vi "DO Close.vi"(8 "error in (no error)":errorcluster, 11 "Mech Pump in":refnum<class "Mech Pump.lvclass">) -> (0 "error out":errorcluster)   [LabVIEW 2021, in "Mech Pump.lvlib" / "Mech Pump.lvclass"]
uses:
  Mech Pump.lvclass
  Mech Pump.lvclass/Mech Pump.ctl
  DAQ-arch/Digital Output On Demand/Digital Output On Demand/Digital Output On Demand.lvclass
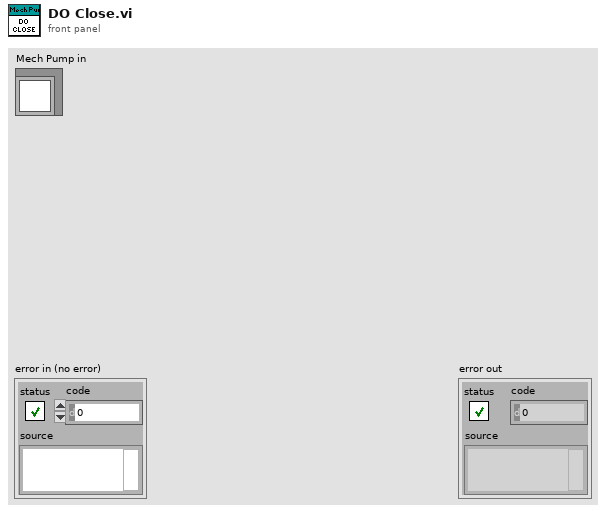
[diagram p1: front panel]
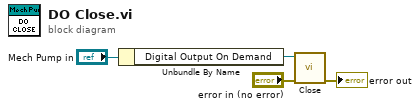
[diagram p0: block diagram]
diagram:
  n1 = Unbundle By Name("Mech Pump in") -> ("Digital Output On Demand"=w3:refnum<class "Digital Output On Demand.lvclass">)
  n2 = call "Close.vi"("error in (no error)"="error in (no error)", "Digital Output On Demand in"=w3) -> ("error out"=→"error out":errorcluster)  [unwired: 9 in]
